vi "Write Data.vi"(10 "Data":i32, 11 "Aquire Data Task Msg in":refnum<class "Aquire Data Task Msg.lvclass">) -> (3 "Aquire Data Task Msg out":refnum<class "Aquire Data Task Msg.lvclass">)   [LabVIEW 2012, in "Aquire Data Actor.lvlib" / "Aquire Data Task Msg.lvclass"]
uses:
  Aquire Data Task Msg.lvclass
  Aquire Data Task Msg.lvclass/Aquire Data Task Msg.ctl
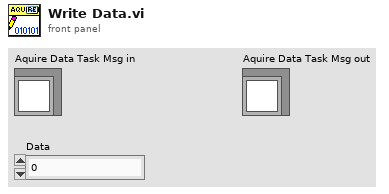
[diagram p1: front panel]
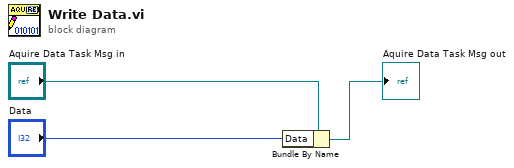
[diagram p0: block diagram]
diagram:
  n1 = Bundle By Name(cluster="Aquire Data Task Msg in", "Data"="Data") -> (→"Aquire Data Task Msg out":refnum<class "Aquire Data Task Msg.lvclass">)
